vi "DateTimeToSQLDT.vi"(10 "DateTimeString":string) -> (2 "SQLDateTime":string)   [LabVIEW 2012]
panel:
  out "x > y?":bool
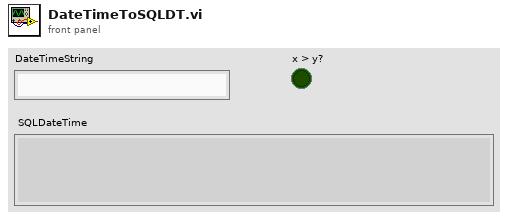
[diagram p1: front panel]
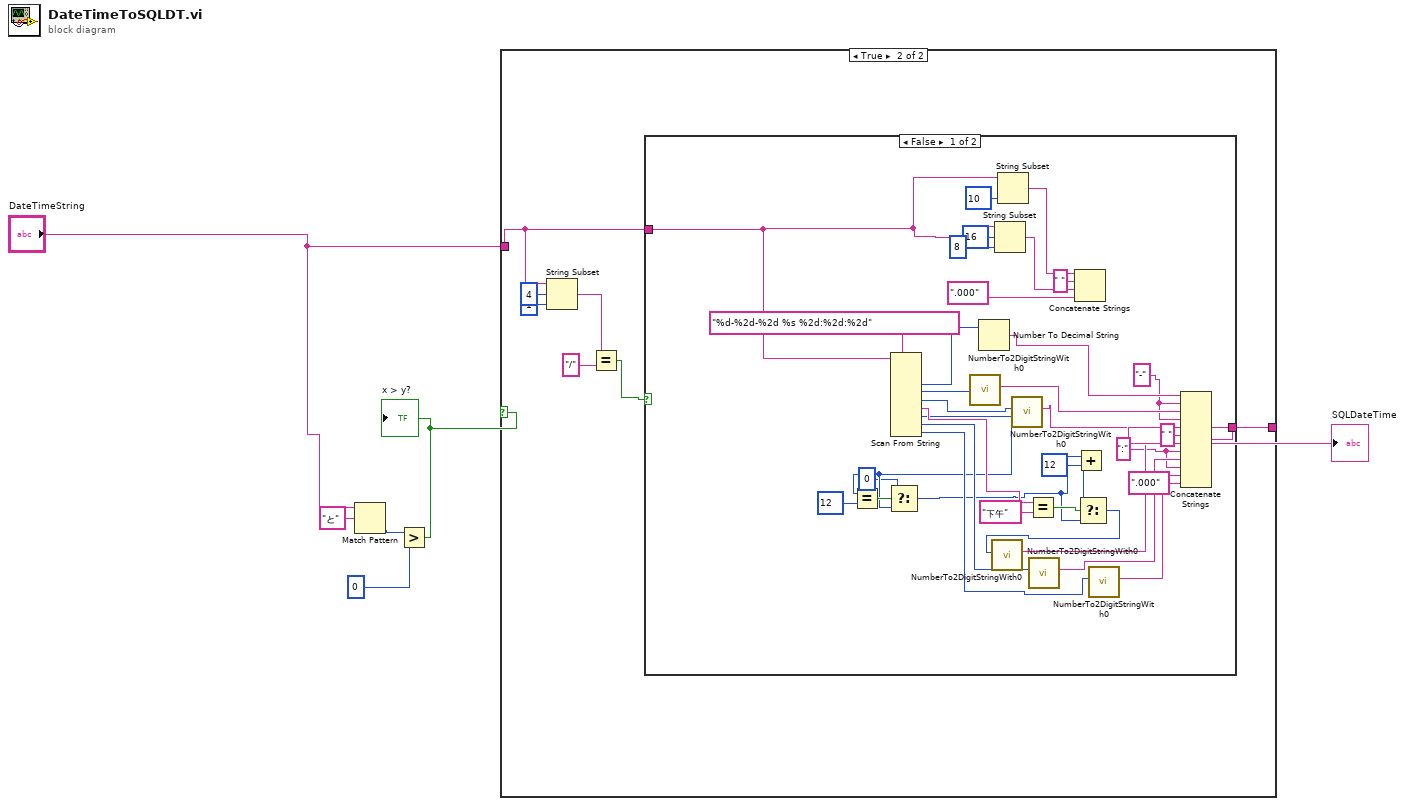
[diagram p0: block diagram]
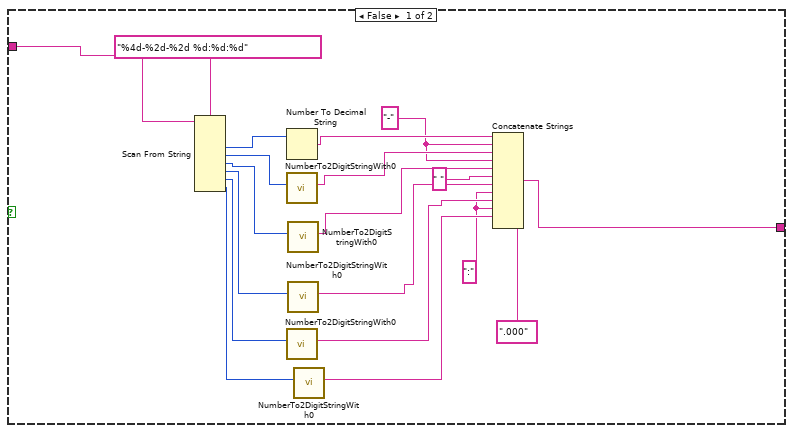
[diagram p2: hidden frame]
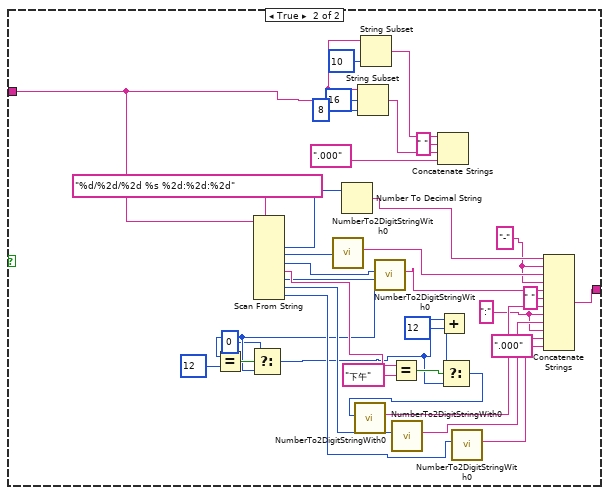
[diagram p3: hidden frame]
diagram:
  n1 = Match Pattern(string="DateTimeString", regular expression="と") -> (offset past match=w4:i32)  [unwired: 1 in, 3 out]
  n2 = Greater?(x=w4, y=0) -> (0:w2:bool)
  "x > y?" <- w2
  n3 = case shown="True" w2 {
    tunnel: [w16 w32] -> w6
    tunnel: "DateTimeString" -> [w25 w26]
    frame False {
      w7 = ":"
      w18 = "-" ("string")
      n4 = Scan From String(format string="%4d-%2d-%2d %d:%d:%d", input string=w25) -> (output 1=w23:i32, output 2=w22:i32, output 3=w21:i32, output 4=w15:i32, output 5=w14:i32, output 6=w13:i32)  [unwired: 8 in, 3 out]
      n5 = Number To Decimal String(number=w23) -> (decimal integer string=w20:string)  [unwired: 1 in]
      n6 = call "NumberTo2DigitStringWith0.vi"("number"=w22) -> ("s? t:f"=w19:string)  [unwired: 10 in]
      n7 = call "NumberTo2DigitStringWith0.vi"("number"=w14) -> ("s? t:f"=w8:string)  [unwired: 10 in]
      n8 = call "NumberTo2DigitStringWith0.vi"("number"=w21) -> ("s? t:f"=w17:string)  [unwired: 10 in]
      n9 = call "NumberTo2DigitStringWith0.vi"("number"=w15) -> ("s? t:f"=w11:string)  [unwired: 10 in]
      n10 = call "NumberTo2DigitStringWith0.vi"("number"=w13) -> ("s? t:f"=w9:string)  [unwired: 10 in]
      n11 = Concatenate Strings(w20, w18, w19, w18, w17, " " ("string"), w11, w7, w8, w7, w9, ".000" ("string")) -> (w16:string)
    }
    frame True {
      n12 = String Subset(string=w26, offset (0)=4, length (rest)=1 ("length (rest)")) -> (substring=w29:string)
      n13 = Equal?(x=w29, y="/") -> (x = y?=w27:bool)
      n14 = case shown="False" w27 {
        tunnel: [w34 w81] -> w32
        tunnel: w26 -> [w33 w69]
        frame False {
          w41 = ":" ("string")
          w43 = "-" ("string")
          n15 = Scan From String(format string="%d-%2d-%2d %s %2d:%2d:%2d", input string=w33) -> (output 1=w61:i32, output 2=w60:i32, output 3=w59:i32, output 4=w56:string, output 5=w38:i32, output 6=w58:i32, output 7=w57:i32)  [unwired: 9 in, 3 out]
          n16 = Equal?(x=w38, y=12) -> (x = y?=w39:bool)
          n17 = Select(t=0, s=w39, f=w38) -> (s? t:f=w36:i32)
          n18 = call "NumberTo2DigitStringWith0.vi"("number"=w60) -> ("s? t:f"=w44:string)  [unwired: 10 in]
          n19 = Number To Decimal String(number=w61) -> (decimal integer string=w45:string)  [unwired: 1 in]
          n20 = String Subset(string=w33, offset (0)=16, length (rest)=8 ("length (rest)")) -> (substring=w63:string)
          n21 = String Subset(string=w33, length (rest)=10 ("length (rest)")) -> (substring=w67:string)  [unwired: 1 in]
          n22 = call "NumberTo2DigitStringWith0.vi"("number"=w59) -> ("s? t:f"=w42:string)  [unwired: 10 in]
          n23 = Equal?(x=w56, y="下午") -> (x = y?=w54:bool)
          n24 = call "NumberTo2DigitStringWith0.vi"("number"=w58) -> ("s? t:f"=w48:string)  [unwired: 10 in]
          n25 = Concatenate Strings(w67, " " ("string"), w63, ".000" ("string")) -> ()  [unwired: 1 out]
          n26 = Add(x=w36, y=12) -> (x+y=w51:i32)
          n27 = Select(t=w51, s=w54, f=w36) -> (s? t:f=w53:i32)
          n28 = call "NumberTo2DigitStringWith0.vi"("number"=w53) -> ("s? t:f"=w49:string)  [unwired: 10 in]
          n29 = call "NumberTo2DigitStringWith0.vi"("number"=w57) -> ("s? t:f"=w47:string)  [unwired: 10 in]
          n30 = Concatenate Strings(w45, w43, w44, w43, w42, " " ("string"), w49, w41, w48, w41, w47, ".000" ("string")) -> (w34:string)
        }
        frame True {
          w76 = ":" ("string")
          w78 = "-" ("string")
          n31 = Scan From String(format string="%d/%2d/%2d %s %2d:%2d:%2d", input string=w69) -> (output 1=w97:i32, output 2=w96:i32, output 3=w95:i32, output 4=w92:string, output 5=w73:i32, output 6=w94:i32, output 7=w93:i32)  [unwired: 9 in, 3 out]
          n32 = Equal?(x=w73, y=12) -> (x = y?=w74:bool)
          n33 = Select(t=0, s=w74, f=w73) -> (s? t:f=w71:i32)
          n34 = call "NumberTo2DigitStringWith0.vi"("number"=w96) -> ("s? t:f"=w79:string)  [unwired: 10 in]
          n35 = Number To Decimal String(number=w97) -> (decimal integer string=w80:string)  [unwired: 1 in]
          n36 = String Subset(string=w69, offset (0)=16, length (rest)=8 ("length (rest)")) -> (substring=w99:string)
          n37 = String Subset(string=w69, length (rest)=10 ("length (rest)")) -> (substring=w103:string)  [unwired: 1 in]
          n38 = call "NumberTo2DigitStringWith0.vi"("number"=w95) -> ("s? t:f"=w77:string)  [unwired: 10 in]
          n39 = Equal?(x=w92, y="下午") -> (x = y?=w90:bool)
          n40 = call "NumberTo2DigitStringWith0.vi"("number"=w94) -> ("s? t:f"=w84:string)  [unwired: 10 in]
          n41 = Concatenate Strings(w103, " " ("string"), w99, ".000" ("string")) -> ()  [unwired: 1 out]
          n42 = Add(x=w71, y=12) -> (x+y=w87:i32)
          n43 = Select(t=w87, s=w90, f=w71) -> (s? t:f=w89:i32)
          n44 = call "NumberTo2DigitStringWith0.vi"("number"=w89) -> ("s? t:f"=w85:string)  [unwired: 10 in]
          n45 = call "NumberTo2DigitStringWith0.vi"("number"=w93) -> ("s? t:f"=w83:string)  [unwired: 10 in]
          n46 = Concatenate Strings(w80, w78, w79, w78, w77, " " ("string"), w85, w76, w84, w76, w83, ".000" ("string")) -> (w81:string)
        }
      }
    }
  }
  "SQLDateTime" <- w6
